vi "Set Or Get NumRows and NumCols.vi"(8 "error in (no error)":errorcluster caption="错误输入（无错误）", 9 "Mode":T1, 10 "Num Rows and cols In":cluster{"NumRows":u32, "NumCols":u32}, 11 "Table Ref In":refnum<vi>) -> (0 "error out":errorcluster caption="错误输出", 2 "Num Rows and cols Out":cluster{"NumRows":u32, "NumCols":u32}, 3 "Table Ref Out":refnum<vi>)   [LabVIEW 2013, in "Table Tool.lvlib"]
uses:
  Table Tool.lvlib
  Custum Type/GetOrSet.ctl
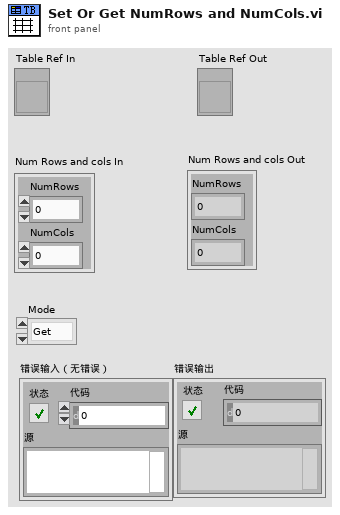
[diagram p1: front panel]
types:
  T1 = typedef "Table Tool.lvlib/GetOrSet.ctl" = enum16{"Get", "Set"}
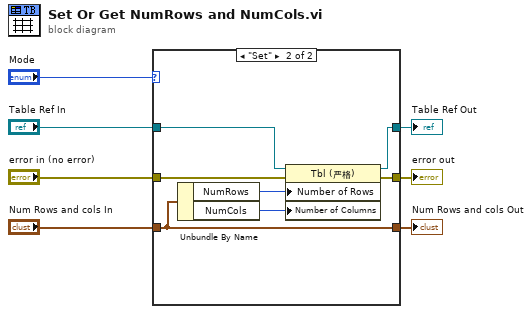
[diagram p0: block diagram]
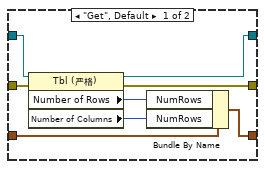
[diagram p2: hidden frame]
diagram:
  n1 = case shown="\"Set\"" "Mode" {
    tunnel: "Table Ref In" -> [w14 w21]
    tunnel: "error in (no error)" -> [w15 w22]
    tunnel: [w12 w19] -> w4
    tunnel: [w13 w20] -> w3
    tunnel: "Num Rows and cols In" -> [w9 w16]
    tunnel: [w8 w16] -> w1
    frame "Get", Default {
      n2 = property class="Tbl (严格)"(reference=w14, error in=w15) -> (reference out=w13:refnum<vi>, error out=w12:errorcluster, "Number of Rows"=w11:u32, "Number of Columns"=w10:u32)
      n3 = Bundle By Name(cluster=w9, "NumRows"=w11, "NumRows"=w10) -> (w8:cluster{"NumRows":u32, "NumCols":u32})
    }
    frame "Set" {
      n4 = Unbundle By Name(w16) -> ("NumRows"=w18:u32, "NumCols"=w17:u32)
      n5 = property class="Tbl (严格)"(reference=w21, error in=w22, "Number of Rows"=w18, "Number of Columns"=w17) -> (reference out=w20:refnum<vi>, error out=w19:errorcluster)
    }
  }
  "Table Ref Out" <- w3
  "error out" <- w4
  "Num Rows and cols Out" <- w1
